vi "FunctionTransformer.vi"(8 "error in (no error)":errorcluster caption="entrée d'erreur (pas d'erreur)", 11 "FunctionTransformer":T1={"func_callable"="None", "inverse_func_callable"="None", "validate"=FALSE, "accept_sparse"=FALSE, "check_inverse"=TRUE, "kw_args"={"key"=[], "Value"=[]}, "inv_kw_args"={"key"=[], "Value"=[]}}) -> (0 "error out":errorcluster, 3 "FunctionTransformer.lvclass":refnum<class "FunctionTransformer.lvclass">)   [LabVIEW 2020]
doc: "Constructs a transformer from an arbitrary callable.\n\nA FunctionTransformer forwards its X (and optionally y) arguments to a user-defined function or function object and returns the result of this function. This is useful for stateless transformations such as taking the log of frequencies, doing custom scaling, etc.\n\nNote: If a lambda is used as the function, then the resulting transformer will not be pickleable.\n\n\n\nParameters : \n\n- func : callable, optional default=None\nThe callable to use for the transformation. This will be passed the same arguments as transform, with args and kwargs forwarded. If func is None, then func will be the identity function.\n\n- inverse_func : callable, optional default=None\nThe callable to use for the inverse transformation. This will be passed the same arguments as inverse transform, with args and kwargs forwarded. If inverse_func is None, then inverse_func will be the identity function.\n\n- validate : bool, optional default=False\nIndicate that the input X array should be checked before calling func. The possibilities are:\n\nIf False, there is no input validation.\n\nIf True, then X will be converted to a 2-dimensional NumPy array or sparse matrix. If the conversion is not possible an exception is raised.\n\n- accept_sparse : boolean, optional\nIndicate that func accepts a sparse matrix as input. If validate is False, this has no effect. Otherwise, if accept_sparse is false, sparse matrix inputs will cause an exception to be raised.\n\n- check_inverse : bool, default=True\nWhether to check that or func followed by inverse_func leads to the original inputs. It can be used for a sanity check, raising a warning when the condition is not fulfilled.\n\n- kw_args : dict, optional\nDictionary of additional keyword arguments to pass to func.\n\n- inv_kw_args : dict, optional\nDictionary of additional keyword arguments to pass to inverse_func.\n\n\nMethods : \n\n\n- Fit : Fit transformer by checking X. If validate is True, X will be checked.\n\nParameters : X : array-like, shape (n_samples, n_features)\n Input array.\n\n- Fit Transform : Fit to data, then transform it. Fits transformer to X and y with optional parameters fit_params and returns a transformed version of X.\n\nParameters : X : {array-like, sparse matrix, dataframe} of shape (n_samples, n_features)\n y : ndarray of shape (n_samples,), default=None\n Target values.\n\nReturns : X_new : ndarray array of shape (n_samples, n_features_new)\n Transformed array.\n\n\n- Transform : Transform X using the forward function.\n\nParameters : X : array-like, shape (n_samples, n_features)\n Input array.\n\nReturns : X_out : array-like, shape (n_samples, n_features)\n Transformed input."
uses:
  FunctionTransformer.lvclass
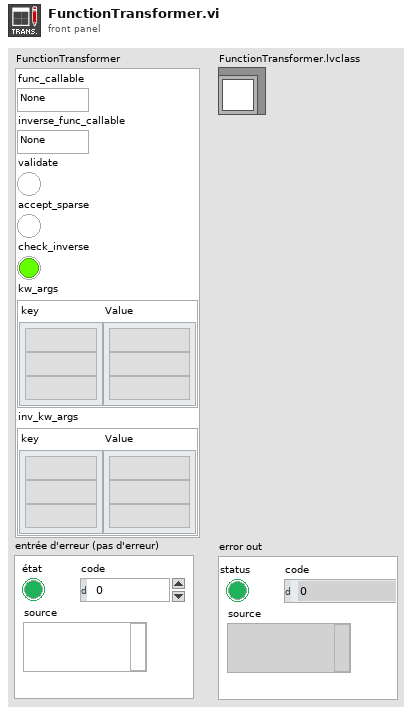
[diagram p1: front panel]
types:
  T1 = cluster{"func_callable":string, "inverse_func_callable":string, "validate":bool, "accept_sparse":bool, "check_inverse":bool, "kw_args":cluster{"key":string[], "Value":string[]}, "inv_kw_args":cluster{"key":string[], "Value":string[]}}
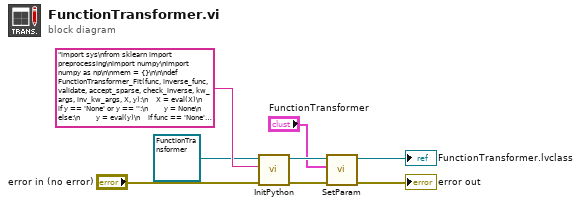
[diagram p0: block diagram]
diagram:
  n1 = call-dynamic "InitPython.vi"("error in (no error)"="error in (no error)", "Python Instruction"="import sys\nfrom sklearn import preprocessing\nimport numpy\nimport numpy as np\n\nmem = {}\n\n\ndef FunctionTransformer_Fit(func, inverse_func, validate, accept_sparse, check_inverse, kw_args, inv_kw_args, X, y):\n    X = eval(X)\n    if y == 'None' or y == '':\n        y = None\n    else:\n        y = eval(y)\n    if func == 'None' or func == '':\n        func = None\n    else :\n        func = eval(func)\n    if inverse_func == 'None' or inverse_func == '':\n        inverse_func = None\n    else :\n        inverse_func = eval(inverse_func)\n    if kw_args == 'None' or kw_args == '':\n        kw_args = None\n    else :\n        kw_args = eval(kw_args)\n    if inv_kw_args == 'None' or inv_kw_args == '':\n        inv_kw_args = None\n    else :\n        inv_kw_args = eval(inv_kw_args)\n    try:\n        FunctionTransformer = preprocessing.FunctionTransformer(func, inverse_func, validate, accept_sparse, check_inverse, kw_args, inv_kw_args).fit(X, y)\n        mem['FitFunctionTransformer'] = FunctionTransformer\n        return str(FunctionTransformer)\n    except:\n        erreur = sys.exc_info()\n        typerr = u\"%s\" % (erreur[0])\n        typerr = typerr[typerr.find(\"'\")+1:typerr.rfind(\"'\")]\n        msgerr = u\"%s\" % (erreur[1])\n        message = str('/!\\\\ {0} : {1}'. format(typerr,msgerr))\n        return message \n    \ndef FunctionTransformer_FitTransform(func, inverse_func, validate, accept_sparse, check_inverse, kw_args, inv_kw_args, X, y):\n    X = eval(X)\n    if y == 'None' or y == '':\n        y = None\n    else:\n        y = eval(y)\n    if func == 'None' or func == '':\n        func = None\n    else :\n        func = eval(func)\n    if inverse_func == 'None' or inverse_func == '':\n        inverse_func = None\n    else :\n        inverse_func = eval(inverse_func)\n    if kw_args == 'None' or kw_args == '':\n        kw_args = None\n    else :\n        kw_args = eval(kw_args)\n    if inv_kw_args == 'None' or inv_kw_args == '':\n        inv_kw_args = None\n    else :\n        inv_kw_args = eval(inv_kw_args)\n    try:\n       \n        FunctionTransformer = preprocessing.FunctionTransformer(func, inverse_func, validate, accept_sparse, check_inverse, kw_args, inv_kw_args).fit_transform(X, y)\n        dtype = type(FunctionTransformer)\n        if dtype == numpy.ndarray:\n            FunctionTransformer = FunctionTransformer.tolist()\n            return str(FunctionTransformer) \n        else:\n            Mat = FunctionTransformer.tocoo()\n            return str(list(zip(Mat.row, Mat.col, Mat.data)))\n    except:\n        erreur = sys.exc_info()\n        typerr = u\"%s\" % (erreur[0])\n        typerr = typerr[typerr.find(\"'\")+1:typerr.rfind(\"'\")]\n        msgerr = u\"%s\" % (erreur[1])\n        message = str('/!\\\\ {0} : {1}'. format(typerr,msgerr))\n        return message \n\ndef FunctionTransformer_Transform(func, inverse_func, validate, accept_sparse, check_inverse, kw_args, inv_kw_args, X, y):\n    X = eval(X)\n    if y == 'None' or y == '':\n        y = None\n    else:\n        y = eval(y)\n    if func == 'None' or func == '':\n        func = None\n    else :\n        func = eval(func)\n    if inverse_func == 'None' or inverse_func == '':\n        inverse_func = None\n    else :\n        inverse_func = eval(inverse_func)\n    if kw_args == 'None' or kw_args == '':\n        kw_args = None\n    else :\n        kw_args = eval(kw_args)\n    if inv_kw_args == 'None' or inv_kw_args == '':\n        inv_kw_args = None\n    else :\n        inv_kw_args = eval(inv_kw_args)\n    try:\n        FunctionTransformer = mem['FitFunctionTransformer'].transform(X)\n        dtype = type(FunctionTransformer)\n        if dtype == numpy.ndarray:\n            FunctionTransformer = FunctionTransformer.tolist()\n            return str(FunctionTransformer) \n        else:\n            Mat = FunctionTransformer.tocoo()\n            return str(list(zip(Mat.row, Mat.col, Mat.data)))\n    except:\n        erreur = sys.exc_info()\n        typerr = u\"%s\" % (erreur[0])\n        typerr = typerr[typerr.find(\"'\")+1:typerr.rfind(\"'\")]\n        msgerr = u\"%s\" % (erreur[1])\n        message = str('/!\\\\ {0} : {1}'. format(typerr,msgerr))\n        return message ", "Scikit-learn en entrée"=refnum<class "FunctionTransformer.lvclass"> refnum ("FunctionTransformer.lvclass")) -> ("error out"=w5:errorcluster, "Scikit-learn en sortie"=w4:refnum<class "FunctionTransformer.lvclass">)  [unwired: 7 in]
  n2 = call-dynamic "SetParam.vi"("error in (no error)"=w5, "FunctionTransformer"="FunctionTransformer", "FunctionTransformer.lvclass"=w4) -> ("error in (no error)"=→"error out":errorcluster, "FunctionTransformer.lvclass"=→"FunctionTransformer.lvclass":refnum<class "FunctionTransformer.lvclass">)  [unwired: 7 in]
